vi "Host - Get Local and ECAT Masters With Retries.vi"(8 "error in (no error)":errorcluster, 11 "serverName":string) -> (0 "error out":errorcluster, 2 "All Local Mods":refnum<k21>[](array[refnum]), 3 "All ECAT Masters":refnum<k21>[](array[refnum]))   [LabVIEW 2019, in "SEECD System Explorer.lvlib"]
uses:
  SEECD System Explorer.lvlib
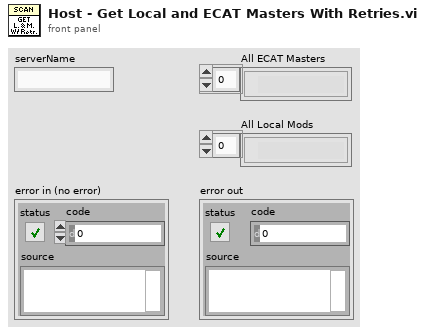
[diagram p1: front panel]
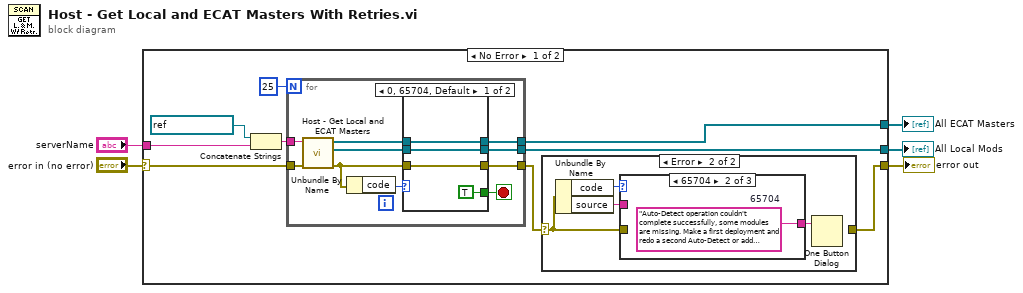
[diagram p0: block diagram]
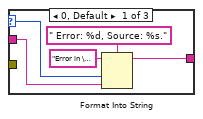
[diagram p3: hidden frame]
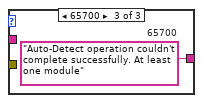
[diagram p4: hidden frame]
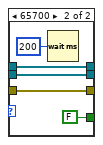
[diagram p5: hidden frame]
diagram:
  n1 = case shown="No Error" "error in (no error)" {
    selector: "error in (no error)" -> [w6 w46]
    tunnel: [w14 w46] -> w5
    tunnel: [w11 _] -> w4
    tunnel: [w9 _] -> w3
    tunnel: "serverName" -> [w8 _]
    frame No Error {
      n2 = Concatenate Strings(refnum<k21> "ni.var.io://" ("IOV Engine in"), w8) -> (w10:string)
      n3 = for {
        N: 25 -> [_]
        tunnel: [w32] -> w9
        tunnel: w10 -> [w35]
        tunnel: [w30] -> w11
        tunnel: w6 -> [w36]
        tunnel: [w28] -> w13
        stop <- w27 stop-if-true
        n4 = call "Host - Get Local and ECAT Masters.vi"("error in (no error)"=w36, "Refnum in"=w35) -> ("error out"=w29:errorcluster, "All Local Mods"=w31:refnum<k21>[], "All ECAT Masters"=w33:refnum<k21>[])  [unwired: 6 in, 1 out]
        n5 = Unbundle By Name(w29) -> ("code"=w34:i32)
        n6 = case shown="0, 65704, Default" w34 {
          tunnel: w33 -> [w40 w45]
          tunnel: [w40 w45] -> w32
          tunnel: w31 -> [w39 w44]
          tunnel: [w39 w44] -> w30
          tunnel: w29 -> [w38 w42]
          tunnel: [w38 w42] -> w28
          tunnel: [TRUE FALSE] -> w27
          frame 0, 65704, Default {
          }
          frame 65700 {
            n7 = Wait (ms)(milliseconds to wait=u32 200) -> ()  [unwired: 1 out]
          }
        }
      }
      n8 = case shown="Error" w13 {
        selector: w13 -> [w15 w18]
        tunnel: [w15 _] -> w14
        frame No Error {
        }
        frame Error {
          n9 = Unbundle By Name(w18) -> ("code"=w19:i32, "source"=w16:string)
          n10 = case shown="65704" w19 {
            selector: w19 -> [w22 _ _]
            tunnel: w18 -> [_ _ _]
            tunnel: [w20 w25 w26] -> w17
            tunnel: w16 -> [w21 _ _]
            frame 0, Default {
              n11 = Format Into String(format string=" Error: %d, Source: %s.", initial string="Error in \"Host - Get Local and ECAT Masters.vi\".", w22, w21) -> (resulting string=w20:string)  [unwired: 1 in, 1 out]
            }
            frame 65704 {
              w25 = "Auto-Detect operation couldn't complete successfully, some modules are missing. Make a first deployment and redo a second Auto-Detect or add manually missing local modules. "  # 65704
            }
            frame 65700 {
              w26 = "Auto-Detect operation couldn't complete successfully. At least one module"  # 65700
            }
          }
          n12 = One Button Dialog(message=w17) -> ()  [unwired: 1 in, 1 out]
        }
      }
    }
    frame Error {
    }
  }
  "error out" <- w5
  "All Local Mods" <- w4
  "All ECAT Masters" <- w3
